vi "Dequeue Broadcast Message by Message Data.vi"(8 "error in (no error)":errorcluster, 9 "Timeout (-1)":i32=-1, 10 "Message Data":variant, 11 "Event Registration Refnum":refnum<event-registration>) -> (0 "error out":errorcluster, 1 "Message Data":variant, 2 "Message":string, 3 "Event Registration Refnum Out":refnum<event-registration>, 4 "Timed Out?":bool)   [LabVIEW 2020, in "Broadcast Event Helpers.lvlib"]
doc: "Dequeue Broadcast messages filtering by message data. The time out for this VI has an error margin of up to one time-out period in edge cases."
uses:
  Broadcast Event Helpers.lvlib
  Process/Protected/Broadcasting/Broadcast Message Cluster.ctl
  Process/Process.lvclass
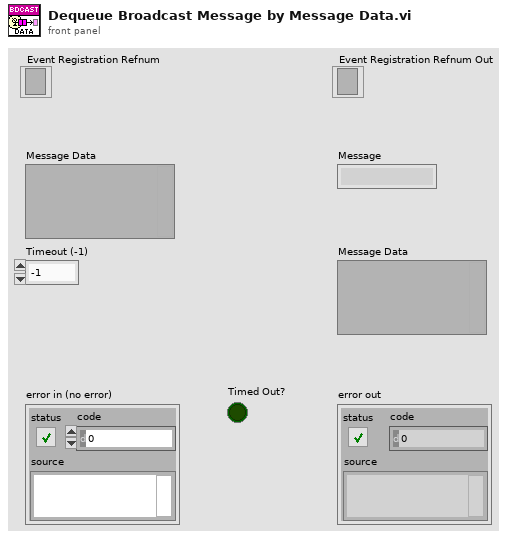
[diagram p1: front panel]
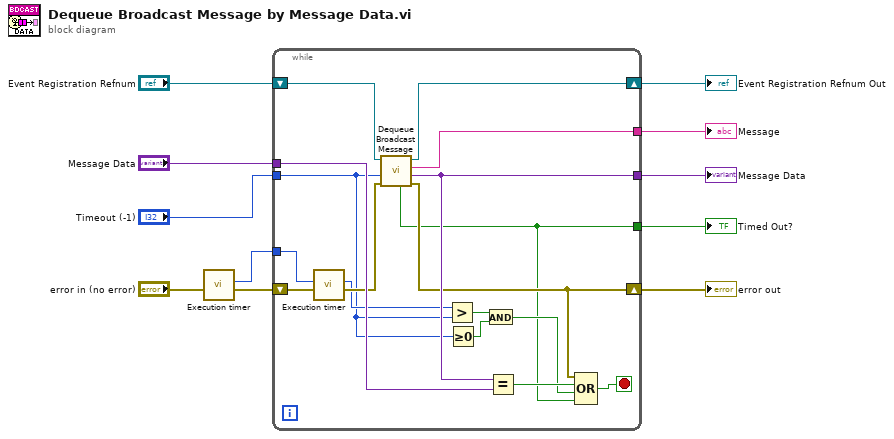
[diagram p0: block diagram]
diagram:
  n1 = call "Execution timer.vi"("error in (no error)"="error in (no error)") -> ("error out"=w2:errorcluster, "Current or Duration [ms]"=w1:u32)  [unwired: 9 in]
  n2 = while {
    tunnel: [w23] -> w7
    tunnel: [w22] -> w6
    tunnel: [w12] -> w5
    tunnel: "Timeout (-1)" -> [w14]
    shift-right: [w27] -> w10
    shift-left: "Event Registration Refnum" -> [w28]
    shift-right: [w20] -> w8
    shift-left: w2 -> [w26]
    tunnel: "Message Data" -> [w25]
    tunnel: w1 -> [w18]
    stop <- w21 stop-if-true
    n3 = call "Execution timer.vi"("error in (no error)"=w26, "millisecond timer value"=w18) -> ("error out"=w19:errorcluster, "Current or Duration [ms]"=w15:u32)  [unwired: 8 in]
    n4 = call "Dequeue Broadcast Message.vi"("error in (no error)"=w19, "Timeout (-1)"=w14, "Event Registration Refnum"=w28) -> ("error out"=w20:errorcluster, "Message Data"=w22:variant, "Message"=w23:string, "Event Registration Refnum Out"=w27:refnum<event-registration>, "Timed Out?"=w12:bool)  [unwired: 3 in, 1 out]
    n5 = Greater?(x=w15, y=w14) -> (0:w17:bool)
    n6 = Greater Or Equal To 0?(x=w14) -> (x >= 0?=w16:bool)
    n7 = And(x=w17, y=w16) -> (x .and. y?=w13:bool)
    n8 = Equal?(x=w22, y=w25) -> (x = y?=w24:bool)
    n9 = Compound Arithmetic op=OR(w20, w24, w13, w12) -> (w21:bool)
  }
  "Event Registration Refnum Out" <- w10
  "Message Data" <- w6
  "Message" <- w7
  "error out" <- w8
  "Timed Out?" <- w5
